vi "SVT Octave Analysis.vi"   [LabVIEW 2017, in "SoundVib_Octave_2014 standard.lvlib"]
doc: "Performs an octave analysis on <B>scaled signal [EU]</B> in accordance with the IEC 61260:2014 and ANSI S1.11-2014 standards. You can use this polymorphic VI to perform octave analysis on a single channel or on N channels. The data type you wire to the <B>scaled signal [EU]</B> input determines the polymorphic instance to use."
uses:
  <vilib>/addons/Sound and Vibration/svt_Octave/SoundVib_Octave_2014 standard.lvlib
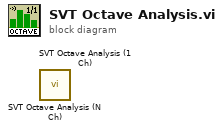
[diagram p0: block diagram]
diagram:
  n1 = call <vilib>:"SVT Octave Analysis (N Ch).vi"() -> ()  [unwired: 10 in, 6 out]
  n2 = call <vilib>:"SVT Octave Analysis (1 Ch).vi"() -> ()  [unwired: 10 in, 6 out]
